vi "Create from Ref.vi"(8 "error in (no error)":errorcluster, 11 "Execution Ref":refnum<k7>) -> (0 "error out":errorcluster, 3 "Execution out":refnum<class "Execution.lvclass">)   [LabVIEW 2020, in "TSnax.lvlib" / "Execution.lvclass"]
uses:
  Execution.lvclass
  Execution.lvclass/Execution.ctl
  Execution Options.ctl
  TSnax.lvlib
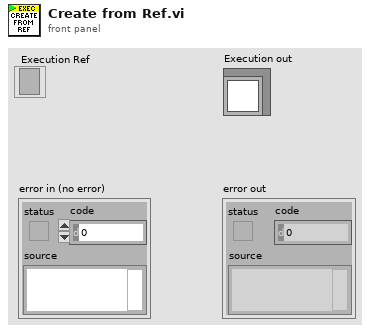
[diagram p1: front panel]
types:
  T1 = typedef "TSnax.lvlib/Execution Options.ctl" = cluster{"Use Default Model (T)":bool, "Release Related References (T)":bool}
  T2 = typedef "TSnax.lvlib/Execution.lvclass/Ref Data.ctl" = cluster{"Parameters":refnum<class "PropertyObject.lvclass">, "Client Sequence":refnum<class "SequenceFile.lvclass">, "Process Model":refnum<class "SequenceFile.lvclass">, "Entry Sequence":string, "Execution":refnum<k7>, "Report":refnum<class "Report.lvclass">, "Options":T1, "Started":bool, "Complete":bool}
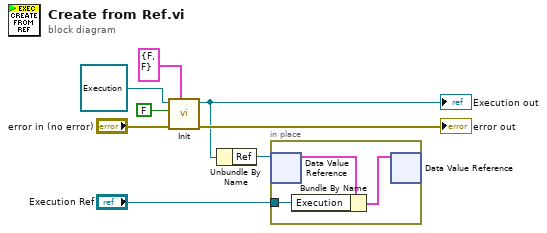
[diagram p0: block diagram]
diagram:
  n1 = call "Init.vi"("Options"=T1 {"Use Default Model (T)"=FALSE, "Release Related References (T)"=FALSE}, "error in (no error)"="error in (no error)", "Daemonized"=FALSE, "Execution in"=refnum<class "Execution.lvclass"> refnum) -> ("error out"=→"error out":errorcluster, "Execution out"=w2:refnum<class "Execution.lvclass">)  [unwired: 6 in]
  "Execution out" <- w2
  n2 = Unbundle By Name(w2) -> ("Ref"=w3:refnum<data-value>)
  n3 = in-place {
    in-place-border: "Execution Ref" -> [w9]
    n4 = in-place-dvr #1(w3) -> (w11:T2)  [unwired: 1 out]
    n5 = Bundle By Name(cluster=w11, "Execution"=w9) -> (w10:T2)
    n6 = in-place-dvr #1(w10) -> ()  [unwired: 2 out]
  }
